vi "Extract_Information.vi"(0 "Input Path":path) -> (1 "File path (Not A Path if cancelled)":path, 2 "Headers":string[](array[string]), 3 "Data Output [V]":dbl[][](array[numeric]), 4 "Error on importing Data":errorcluster)   [LabVIEW 2023]
doc: "This simple VI is used to import the data from a .csv file, under the hypothesis that the delimiter is a \",\".\nThe used functions automatically close the file, once read.\nInputs:\n- Filepath\nOutputs:\n- Filepath\n- Headers for visualisation\n- Datas\n- Error on importing Data"
uses:
  <vilib>/Utility/file.llb/Read Delimited Spreadsheet (DBL).vi
  <vilib>/Utility/file.llb/Read Delimited Spreadsheet (string).vi
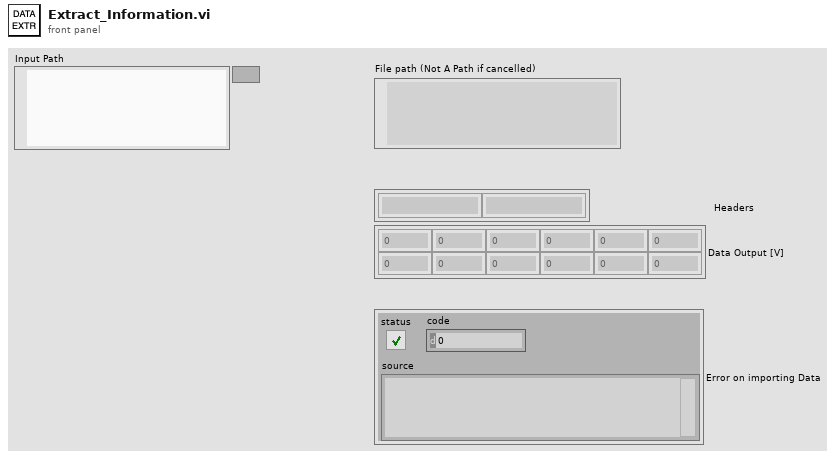
[diagram p1: front panel]
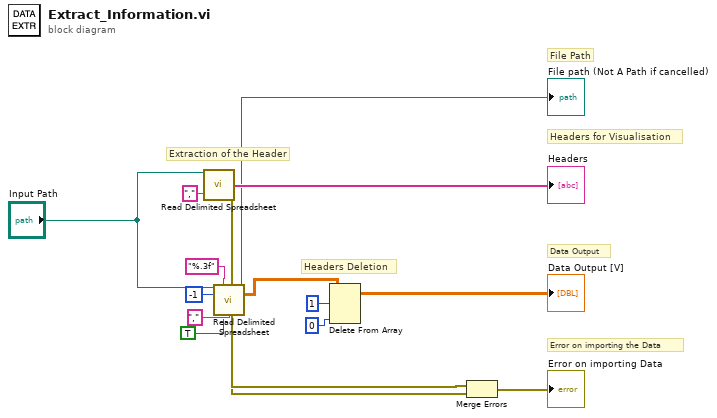
[diagram p0: block diagram]
diagram:
  # "File Path"
  # "Error on importing the Data"
  # "Extraction of the Header"
  # "Data Output"
  # "Headers for Visualisation"
  # "Headers Deletion"
  n1 = call-poly <vilib>:"Read Delimited Spreadsheet.vi"("file path (dialog if empty)"="Input Path", "delimiter (\\t)"="," ("delimiter (\\t)")) -> ("first row"=→"Headers":string[], "error out"=w3:errorcluster)  [unwired: 8 in, 4 out]
  n2 = call-poly <vilib>:"Read Delimited Spreadsheet.vi"("file path (dialog if empty)"="Input Path", "format (%.3f)"="%.3f", "number of rows (all:-1)"=-1, "transpose? (F)"=TRUE, "delimiter (\\t)"="," ("delimiter (\\t)")) -> ("new file path (Not A Path if cancelled)"=→"File path (Not A Path if cancelled)":path, "all rows"=w12:dbl[][], "error out"=w4:errorcluster)  [unwired: 5 in, 3 out]
  n3 = Delete From Array(array=w12, length=1 ("index"), index (col)=0 ("index")) -> (array with subset deleted=→"Data Output [V]":dbl[][])  [unwired: 1 in, 1 out]
  n4 = Merge Errors(w4, w3) -> (→"Error on importing Data":errorcluster)
